vi "Main.vi"(8 "error in (no error)":errorcluster, 11 "ModuleAdmin":refnum<class "ModuleAdmin.lvclass">) -> ()   [LabVIEW 2018, in "DigitizerPlugins.lvlib"]
uses:
  DigitizerPlugins.lvlib
  <userlib>/NIST/ModuleAdminLib/ModuleAdmin/ModuleAdmin.lvclass
  C:/Program Files/National Instruments/LabVIEW 2018/user.lib/NIST/ModuleAdminLib/ModuleAdminBase/ModuleAdminBase.lvclass
  DigitizerShared/clStopArgument.ctl
  DigitizerBaseClass/DigitizerBase.lvclass
  C:/Program Files/National Instruments/LabVIEW 2018/user.lib/NIST/BaseClasses/BasePlugin_class/BasePlugin.lvclass
  <userlib>/NIST/ModuleAdminLib/ModuleAdmin/ModuleAdmin.lvclass/ModuleAdmin.ctl
  <userlib>/NIST/BaseClasses/BasePlugin_class/BasePlugin.lvclass/BasePlugin.ctl
  DigitizerBaseClass/DigitizerBase.lvclass/DigitizerBase.ctl
  DigitizerBaseClass/Typedefs/Channel.ctl
  DigitizerBaseClass/Typedefs/Acquisition.ctl
  DigitizerBaseClass/Typedefs/Trigger.ctl
  DigitizerBaseClass/Typedefs/TrigSource.ctl
  <vilib>/Utility/error.llb/DialogType.ctl
  <userlib>/NIST/ModuleAdminLib/ModuleAdmin/Accessors/Read ShowPanel_.vi
  <userlib>/NIST/ModuleAdminLib/ModuleAdmin/Accessors/Write ShowPanel_.vi
  <userlib>/NIST/BaseClasses/BasePlugin_class/Accessors/Write PluginIniFilePath.vi
  <userlib>/NIST/BaseClasses/BasePlugin_class/Accessors/Read PluginIniFilePath.vi
  DigitizerBaseClass/Accessors/Read Channels.vi
  DigitizerBaseClass/Accessors/Write Channels.vi
  DigitizerBaseClass/Accessors/Read Acquisition.vi
  DigitizerBaseClass/Accessors/Write Acquisition.vi
  DigitizerBaseClass/Accessors/Read Trigger.vi
  DigitizerBaseClass/Accessors/Write Trigger.vi
  DigitizerBaseClass/Accessors/Read Waveforms.vi
  <userlib>/NIST/ModuleAdminLib/ModuleAdmin/Accessors/Read CloneRegRef.vi
  <extravilib>/ChannelInstances/Tag-bool/Read With Abort.vi
  <extravilib>/ChannelInstances/Tag-bool/Write With Abort.vi
  <extravilib>/ChannelInstances/Tag-bool/Instantiate.vi
  <extravilib>/ChannelInstances/Tag-bool/EndpointRead.vi
  <vilib>/Utility/error.llb/Error Cluster From Error Code.vi
  <extravilib>/ChannelInstances/Tag-bool/Endpoint.vi
  <vilib>/ErrorRing/Error Ring.xnode
  <userlib>/NIST/ModuleAdminLib/CloneRegistration/CloneRegistration.lvclass
  DigitizerShared/DigitizerShared.lvlib
  <userlib>/NIST/BaseClasses/Object_class/BaseObject.lvclass
  <userlib>/NIST/ModuleAdminLib/ModuleAdmin.lvlib
  <extravilib>/ChannelInstances/Tag-bool.lvlib
panel:
  out "error out":errorcluster
  # "This is the template for your cloneable module.\nYou should modifiy this to perform the functionality\nthat you want it to perform"
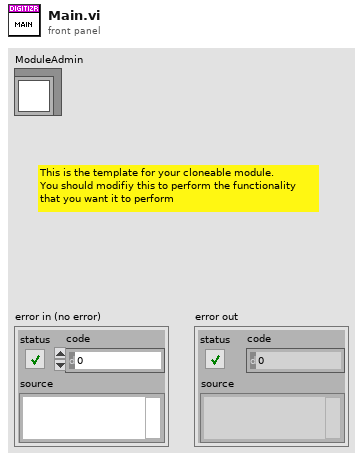
[diagram p1: front panel]
types:
  T1 = typedef "DigitizerShared.lvlib/clRequestEvents.ctl" = cluster{"StopRequest":refnum<user-event>, "PathToINI":refnum<user-event>, " LoadPlugin":refnum<user-event>, "ShowPanel":refnum<user-event>, "PrefDlg":refnum<user-event>, "ReadChannels":refnum<user-event>, "WriteChannels":refnum<user-event>, "ConfigChannels":refnum<user-event>, "ReadAcq":refnum<user-event>, "WriteAcq":refnum<user-event>, "ConfigAcq":refnum<user-event>, "ReadTriggers":refnum<user-event>, "WriteTriggers":refnum<user-event>, "ConfigTriggers":refnum<user-event>, "FetchWfrm":refnum<user-event>, "ReadWfrm":refnum<user-event>, "Initialize":refnum<user-event>, "Abort":refnum<user-event>, "ReadSyncInfo":refnum<user-event>, "WriteSyncInfo":refnum<user-event>, "Close":refnum<user-event>}
  T2 = typedef "DigitizerShared.lvlib/clBroadcastEvents.ctl" = cluster{"DidInit":refnum<user-event>, "StatusUpdate":refnum<user-event>, "ErrorReport":refnum<user-event>, "DidStop":refnum<user-event>, "PathToINI":refnum<user-event>, "Channels":refnum<user-event>, "Acq":refnum<user-event>, "Trigger":refnum<user-event>, "Waveforms":refnum<user-event>}
  T3 = typedef "DigitizerShared.lvlib/clStopArgument.ctl" = cluster{"Exit via Stop Module Req?":bool, "Wait for Module to stop?":bool, "ModuleAdmin":refnum<class "ModuleAdmin.lvclass">}
  T4 = enum32{"Invalid", "Standard", "Closed", "Hidden", "Minimized", "Maximized"}
  T5 = typedef "DigitizerPlugins.lvlib/DigitizerBase.lvclass/Channel.ctl" = cluster{"Name":string, "Enabled":bool, "InputImpedance":dbl, "Coupling":enum16{"AC", "DC", "Gnd"}, "Offset":dbl, "Range":dbl}
  T6 = typedef "DigitizerPlugins.lvlib/DigitizerBase.lvclass/Acquisition.ctl" = cluster{"SampleRate":dbl, "RecordSize":i32, "NumRecords":i32, "SampleMode":i32, "Timeout (ms)":i32}
  T7 = typedef "DigitizerPlugins.lvlib/DigitizerBase.lvclass/Trigger.ctl" = cluster{"Source":string, "Delay":dbl, "Holdoff":dbl, "PretriggerSamples":i32, "Sources":T8[]}
  T8 = typedef "DigitizerPlugins.lvlib/DigitizerBase.lvclass/TrigSource.ctl" = cluster{"Name":string, "Coupling":enum16{"AC", "DC", "HF Reject", "LF Reject", "Noise Reject"}, "Hysteresis":dbl, "Level":dbl, "Slope":enum16{"Positive", "Negative"}, "Type":enum16{"Edge", "Width", "Runt", "Glitch", "TV", "Window"}}
  T9 = typedef "Tag-bool.lvlib/))Channel.ctl" = refnum<queue>
  T10 = typedef "DialogType.ctl" = u16
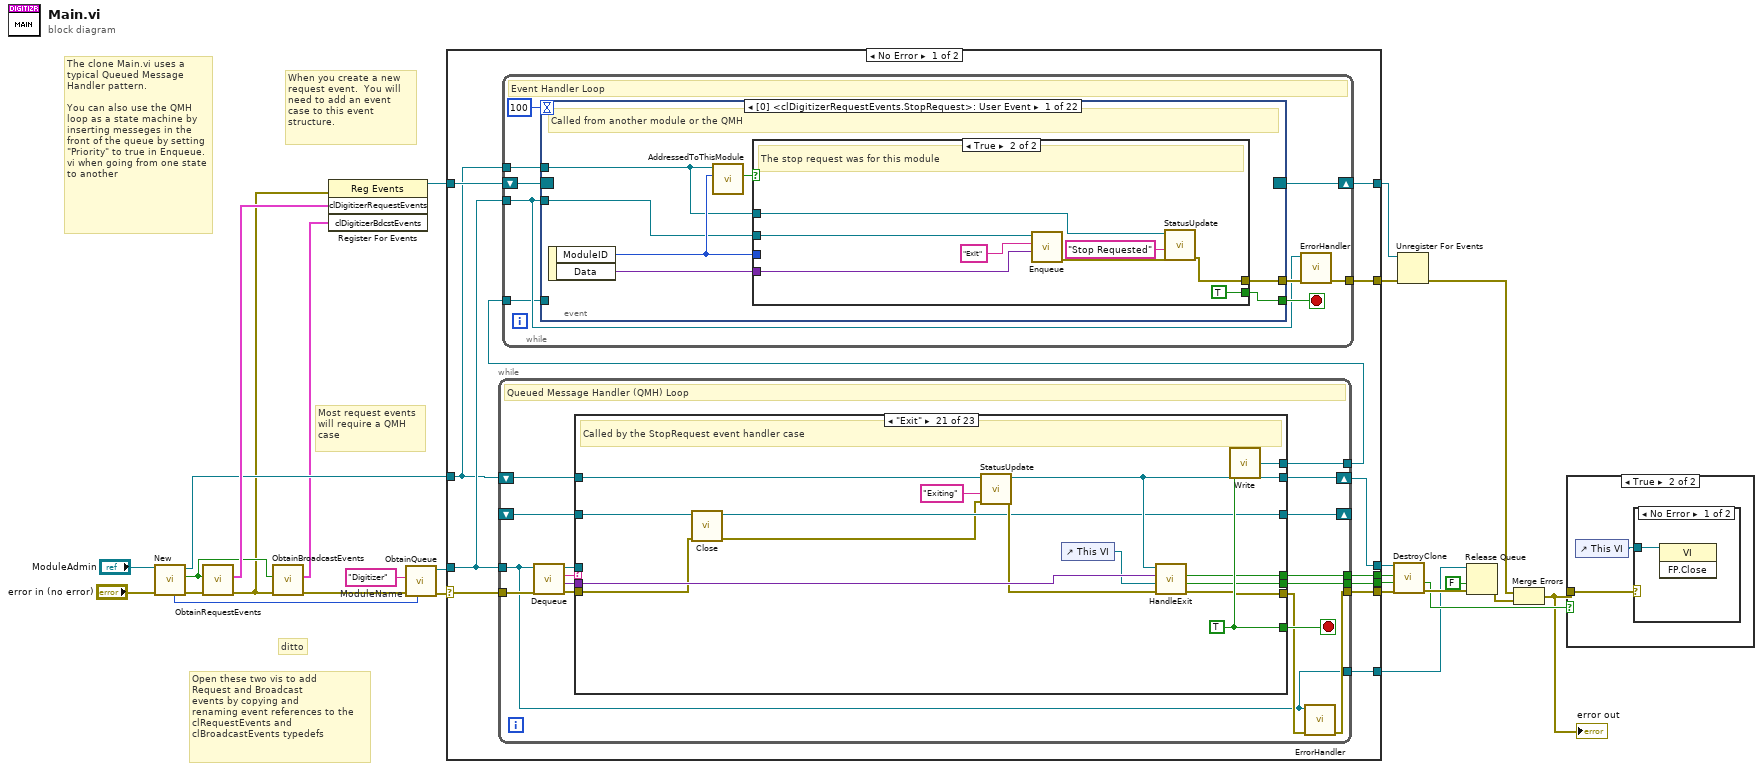
[diagram p0: block diagram]
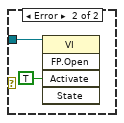
[diagram p3: hidden frame]
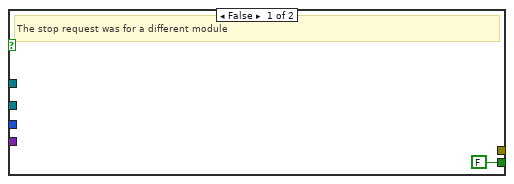
[diagram p4: hidden frame]
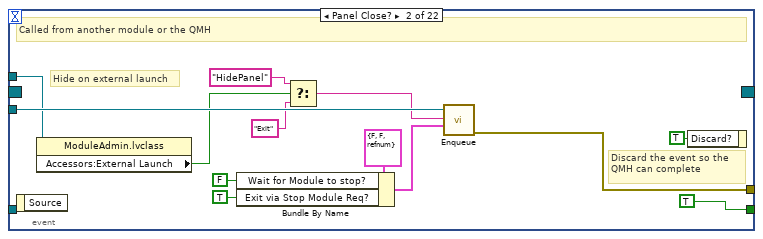
[diagram p5: hidden frame]
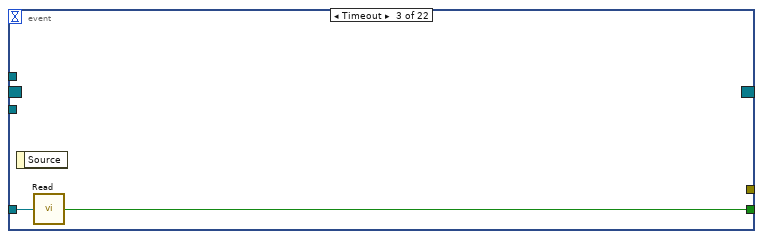
[diagram p6: hidden frame]
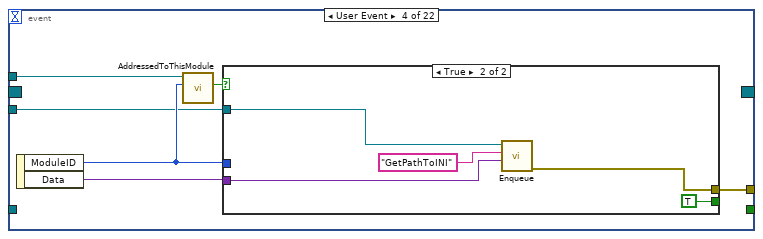
[diagram p7: hidden frame]
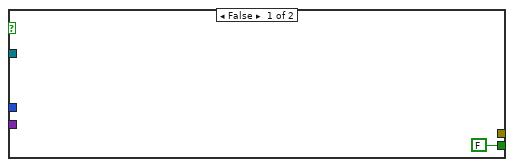
[diagram p8: hidden frame]
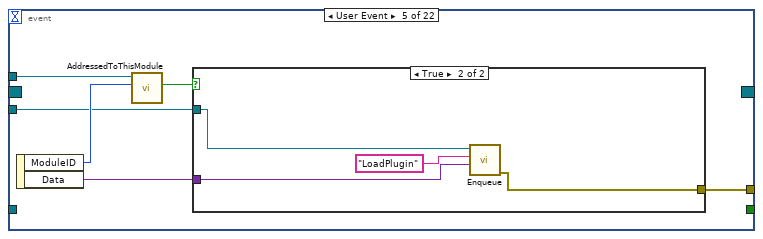
[diagram p9: hidden frame]
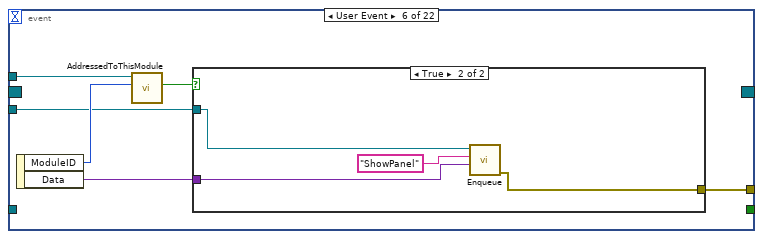
[diagram p11: hidden frame]
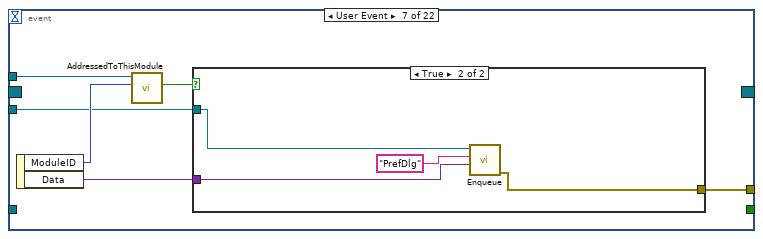
[diagram p13: hidden frame]
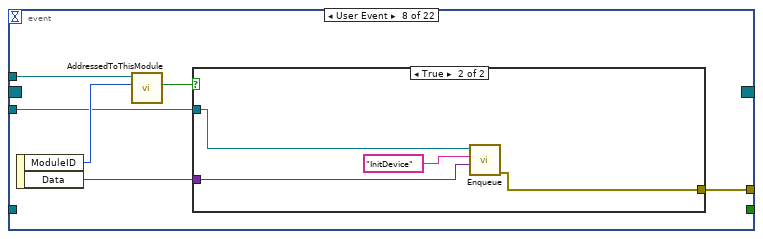
[diagram p15: hidden frame]
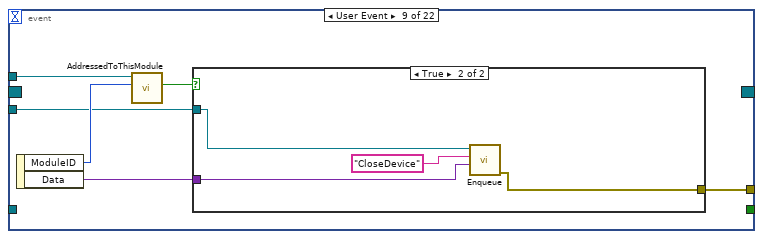
[diagram p17: hidden frame]
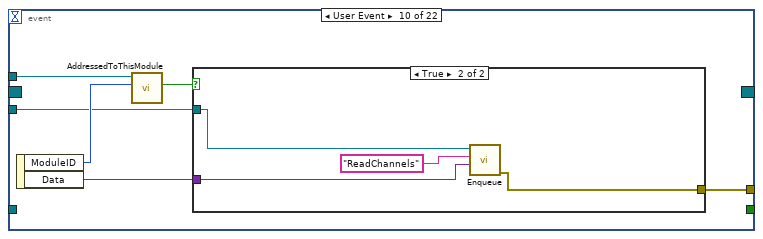
[diagram p19: hidden frame]
diagram:
  w1 = "Digitizer"  # ModuleName
  # "The clone Main.vi uses a typical Queued Message Handler pattern.  \n\nYou can also use the QMH loop as a state machine by inserting messeges in the front of the queue by setting \"Priority\" to true in Enqueue.vi when going from one state to another"
  # "Open these two vis to add\nRequest and Broadcast \nevents by copying and \nrenaming event references to the \nclRequestEvents and \nclBroadcastEvents typedefs"
  # "ditto"
  # "Most request events\nwill require a QMH\ncase"
  # "When you create a new request event.  You will need to add an event case to this event structure."
  n1 = call <userlib>:"New.vi"("error in (no error)"="error in (no error)", "ModuleAdmin"="ModuleAdmin") -> ("error out"=w25:errorcluster, "First?"=w19:bool, "ModuleAdmin"=w21:refnum<class "ModuleAdmin.lvclass">, "Module ID"=w2:i32)  [unwired: 6 in]
  n2 = call "ObtainRequestEvents.vi"("error in (no error)"=w25, "CreateNew (F)"=w19) -> ("error out"=w18:errorcluster, "clDigitizerRequestEvents"=w24:T1)  [unwired: 8 in]
  n3 = call "ObtainBroadcastEvents.vi"("error in (no error)"=w18, "CreateNew? (F)"=w19) -> ("error out"=w20:errorcluster, "clDigitizerBdcstEvents"=w17:T2)  [unwired: 8 in]
  n4 = register-events(error in=w18, w24, w17) -> (reference out=w16:refnum<event-registration>)  [unwired: 1 in, 1 out]
  n5 = call "ObtainQueue.vi"("ModuleID"=w2, "error in (no error)"=w20, "ModuleName"=w1) -> ("error out"=w23:errorcluster, "MessageQueue"=w22:refnum<queue>)  [unwired: 7 in]
  n6 = case shown="No Error" w23 {
    selector: w23 -> [w39 w631]
    tunnel: w22 -> [w37 w623]
    tunnel: w21 -> [w35 w628]
    tunnel: [w38 w629] -> w15
    tunnel: w16 -> [w36 w624]
    tunnel: [w34 w627] -> w13
    tunnel: [w33 _] -> w12
    tunnel: [w32 _] -> w11
    tunnel: [w31 _] -> w8
    tunnel: [w30 w624] -> w7
    tunnel: [w29 w623] -> w4
    frame No Error {
      n7 = while {
        tunnel: w37 -> [w274]
        tunnel: w39 -> [w286]
        tunnel: [w279] -> w38
        tunnel: [w281] -> w33
        tunnel: [w280] -> w32
        shift-right: [w277] -> _
        shift-left: _ -> [w276]
        shift-right: [w275] -> w34
        shift-left: w35 -> [w282]
        tunnel: [w274] -> w29
        tunnel: [w273] -> w28
        stop <- w287 stop-if-true
        # "Queued Message Handler (QMH) Loop"
        n8 = call "Dequeue.vi"("error in (no error)"=w286, "MessageQueue"=w274) -> ("error out"=w285:errorcluster, "Message Data"=w283:variant, "Message"=w284:string, "MessageQueue"=w272:refnum<queue>)  [unwired: 6 in]
        n9 = case shown="\"Exit\"" w284 {
          selector: w284 -> [_ _ _ _ _ _ _ _ _ _ _ _ _ _ _ _ _ _ _ _ _ _ w611]
          tunnel: [_ _ _ _ _ _ _ _ _ _ _ _ _ _ _ _ _ _ _ _ w581 _ _] -> w287
          tunnel: w282 -> [w308 w325 w333 w380 w383 w394 w399 w414 w428 w433 w448 w462 w467 w484 w491 w502 w517 w530 w546 w558 w575 w585 w614]
          tunnel: [w297 w318 w334 w381 w386 w388 w396 w408 w423 w430 w442 w457 w464 w481 w485 w500 w515 w521 w537 w553 w580 w586 w610] -> w278
          tunnel: w285 -> [_ w328 w343 w376 w387 w392 w406 w411 w427 w440 w443 w461 w474 w478 w488 w504 w519 w528 w543 w557 w569 w594 _]
          tunnel: w283 -> [_ w327 w345 _ _ _ w407 _ _ w441 _ _ w475 w479 _ _ _ _ _ _ w579 w593 _]
          tunnel: [_ _ _ _ _ _ _ _ _ _ _ _ _ _ _ _ _ _ _ _ w577 _ _] -> w281
          tunnel: [_ _ _ _ _ _ _ _ _ _ _ _ _ _ _ _ _ _ _ _ w576 _ _] -> w280
          tunnel: [refnum<class "DigitizerBase.lvclass"> refnum ("MyPlugins.lvlib:MyPluginsBase.lvclass") w317 w331 w377 w384 w390 w402 w409 w425 w436 w445 w459 w470 w477 w486 w501 w516 w523 w541 w555 w570 w584 w608] -> w277
          tunnel: w276 -> [_ w317 w332 w379 w385 w395 w404 w412 w429 w438 w446 w463 w472 w480 w489 w505 w520 w526 w545 w556 w571 w584 w608]
          tunnel: [w288 w324 w329 w374 w383 w389 w398 w413 w424 w432 w447 w458 w466 w483 w490 w499 w514 w522 w539 w559 w574 w583 w607] -> w275
          tunnel: [_ _ _ _ _ _ _ _ _ _ _ _ _ _ _ _ _ _ _ _ w567 _ _] -> w273
          tunnel: w272 -> [_ _ _ _ _ _ _ _ _ _ _ _ _ _ _ _ _ _ _ _ _ w582 _]
          frame "Initialize" {
            # "Initialize is always called after ObtainQueue.vi is run"
            n10 = property class="ModuleAdmin.lvclass"(reference=w308) -> (reference out=w294:refnum<class "ModuleAdmin.lvclass">, error out=w305:errorcluster, "Accessors:Module ID"=w296:i32, "Accessors:ShowPanel_"=w291:bool, "Accessors:External Launch"=w290:bool, "Accessors:ModuleName"=w292:string)  [unwired: 1 in]
            n11 = Compound Arithmetic op=OR(w291, invert w290) -> (w289:bool)
            n12 = Select(t=T4."Standard" ("Front Panel Window:State"), s=w289, f=T4."Hidden" ("Front Panel Window:State")) -> (s? t:f=w301:T4)
            n13 = invoke class="VI" method="FP.Open"(error in=w305, "State"=w301) -> (error out=w304:errorcluster)  [unwired: 3 in, 4 out]
            n14 = call <userlib>:"ModuleName.vi"("Name"=w292, "ModuleID"=w296) -> ("ModuleName"=w300:string)  [unwired: 9 in]
            n15 = property class="VI"(error in=w304, "Front Panel.Title"=w300) -> (reference out=w307:refnum<vi>, error out=w306:errorcluster)  [unwired: 1 in]
            n16 = invoke class="VI" method="FP.Center"(reference=w307, error in=w306) -> (error out=w295:errorcluster)  [unwired: 1 in, 2 out]
            n17 = case shown="True" w290 {
              tunnel: [w309 w315] -> w298
              tunnel: [w310 w312] -> w288
              tunnel: w295 -> [w309 w314]
              tunnel: w294 -> [w310 w311]
              frame False {
              }
              frame True {
                n18 = call <userlib>:"WaitOnModuleSync.vi"("error in (no error)"=w314, "ModuleAdmin"=w311) -> ("error out"=w316:errorcluster, "ModuleAdmin"=w313:refnum<class "ModuleAdmin.lvclass">)  [unwired: 8 in]
                n19 = call <userlib>:"WaitOnEventSync.vi"("error in (no error)"=w316, "ModuleAdmin"=w313) -> ("error out"=w315:errorcluster, "ModuleAdmin"=w312:refnum<class "ModuleAdmin.lvclass">)  [unwired: 8 in]
              }
            }
            n20 = call "DidInit.vi"("Init?"=TRUE, "error in (no error)"=w298, "ModuleAdmin"=w288) -> ("error out"=w297:errorcluster)  [unwired: 8 in]
          }
          frame "ShowPanel" {
            # "The frontpanel can be shown or hidden"
            n21 = Variant To Data(error in=w328, type=TRUE, Variant=w327) -> (data=w320:bool, error out=w323:errorcluster)
            n22 = Select(t=T4."Standard" ("Front Panel Window:State"), s=w320, f=T4."Hidden" ("Front Panel Window:State")) -> (s? t:f=w319:T4)
            n23 = property class="VI"(error in=w323, "FP.State"=w319) -> (error out=w318:errorcluster)  [unwired: 1 in, 1 out]
            n24 = property class="ModuleAdmin.lvclass"(reference=w325, "Accessors:ShowPanel_"=w320) -> (reference out=w324:refnum<class "ModuleAdmin.lvclass">)  [unwired: 1 in, 1 out]
          }
          frame "LoadPlugin" {
            # "Dynamically oads and initializes a plugin from the .ini file"
            n25 = Variant To Data(error in=w343, type=path "", Variant=w345) -> (data=w330:path, error out=w342:errorcluster)
            n26 = call <userlib>:"GetPathToClass.vi"("error in (no error)"=w342, "configuration file path"=w330) -> ("error IO"=w338:errorcluster, "PathToClass"=w341:path)  [unwired: 8 in]
            n27 = Current VI's Path() -> (path=w340:path)
            n28 = Build Path(base path=w340, name or relative path=w341) -> (appended path=w339:path)
            n29 = call <vilib>:"Check if File or Folder Exists.vi"("error in (no error)"=w338, "path"=w339) -> ("error out"=w335:errorcluster, "file or folder exists?"=w337:bool, "dup path"=w336:path)  [unwired: 7 in]
            n30 = case shown="True" w337 {
              tunnel: w336 -> [w349 w366]
              tunnel: w335 -> [_ w373]
              tunnel: [w348 w368] -> w334
              tunnel: w333 -> [w346 w363]
              tunnel: w332 -> [w347 _]
              tunnel: [w347 w359] -> w331
              tunnel: w330 -> [_ w364]
              tunnel: [w346 w362] -> w329
              frame False {
                n31 = Path To String(path=w349) -> (string=w350:string)
                n32 = xnode "Error Ring"("parameter 0"=w350) -> ("error out"=w348:errorcluster)
              }
              frame True {
                n33 = call-dynamic "LoadClassFromFile.vi"("error in (no error)"=w373, "class path"=w366, "reference in"=refnum<class "DigitizerBase.lvclass"> refnum ("MyPlugins.lvlib:MyPluginsBase.lvclass")) -> ("error out"=w365:errorcluster, "reference out"=w367:refnum<class "DigitizerBase.lvclass">)  [unwired: 7 in]
                n34 = property class="DigitizerBase.lvclass"(reference=w367, error in=w365, "Accessors:PluginIniFilePath"=w364) -> (reference out=w361:refnum<class "DigitizerBase.lvclass">, error out=w360:errorcluster)
                n35 = Path To String(path=w366) -> (string=w370:string)
                n36 = Format Into String(format string="Plugin %s loaded ", w370) -> (resulting string=w369:string)  [unwired: 2 in, 1 out]
                n37 = call-dynamic "DefaultFromIni.vi"("error in (no error)"=w360, "MyPluginsBase in"=w361) -> ("error out"=w358:errorcluster, "MyPluginsBase out"=w359:refnum<class "DigitizerBase.lvclass">)  [unwired: 8 in]
                n38 = call "StatusUpdate.vi"("error in (no error)"=w358, "Status"=w369, "Module"=w363) -> ("error out"=w368:errorcluster, "Module"=w362:refnum<class "ModuleAdmin.lvclass">)  [unwired: 7 in]
              }
            }
          }
          frame "GetPathToINI" {
            # "Broadcast the path to the .ini file"
            n39 = property class="DigitizerBase.lvclass"(reference=w379, error in=w376) -> (reference out=w377:refnum<class "DigitizerBase.lvclass">, error out=w375:errorcluster, "Accessors:PluginIniFilePath"=w378:path)
            n40 = property class="ModuleAdmin.lvclass"(reference=w380) -> (reference out=w374:refnum<class "ModuleAdmin.lvclass">, "Accessors:Module ID"=w382:i32)  [unwired: 1 in, 1 out]
            n41 = call "PathToINIBroadcast.vi"("error in (no error)"=w375, "PathToINI"=w378, "ModuleID"=w382) -> ("error out"=w381:errorcluster)  [unwired: 8 in]
          }
          frame "PrefDlg" {
            # "Override Base Class\\PublicMethods\\PrefDialog.vi for user editable preference dialog"
            # "Launch the modal Preferences dialog"
            n42 = call-dynamic "PrefDialog.vi"("error in (no error)"=w387, "DigitizerBase"=w385) -> ("error out"=w386:errorcluster, "DigitizerBase"=w384:refnum<class "DigitizerBase.lvclass">)  [unwired: 8 in]
          }
          frame "ReadChannels" {
            n43 = property class="DigitizerBase.lvclass"(reference=w395, error in=w392) -> (reference out=w390:refnum<class "DigitizerBase.lvclass">, error out=w391:errorcluster, "Accessors:Channels"=w393:T5[])
            n44 = call "ChannelBdcst.vi"("error in (no error)"=w391, "Channels"=w393, "Module"=w394) -> ("error out"=w388:errorcluster, "Module"=w389:refnum<class "ModuleAdmin.lvclass">)  [unwired: 7 in]
          }
          frame "WriteChannels" {
            n45 = Variant To Data(error in=w406, type=T5[] [], Variant=w407) -> (data=w403:T5[], error out=w401:errorcluster)
            n46 = property class="DigitizerBase.lvclass"(reference=w404, error in=w401, "Accessors:Channels"=w403) -> (reference out=w402:refnum<class "DigitizerBase.lvclass">, error out=w400:errorcluster)
            n47 = call "StatusUpdate.vi"("error in (no error)"=w400, "Status"="Received Channels", "Module"=w399) -> ("error out"=w396:errorcluster, "Module"=w398:refnum<class "ModuleAdmin.lvclass">)  [unwired: 7 in]
          }
          frame "ConfigChannels" {
            n48 = call-dynamic "ConfigChannels.vi"("error in (no error)"=w411, "DigitizerBase in"=w412) -> ("error out"=w410:errorcluster, "DigitizerBase out"=w409:refnum<class "DigitizerBase.lvclass">)  [unwired: 8 in]
            n49 = case shown="No Error" w410 {
              selector: w410 -> [w419 w420]
              tunnel: w414 -> [w418 w421]
              tunnel: [w416 w420] -> w408
              tunnel: [w415 w421] -> w413
              frame No Error {
                n50 = call "StatusUpdate.vi"("error in (no error)"=w419, "Status"="Channels Configured", "Module"=w418) -> ("error out"=w416:errorcluster, "Module"=w415:refnum<class "ModuleAdmin.lvclass">)  [unwired: 7 in]
              }
              frame Error {
              }
            }
          }
          frame "ReadAcq" {
            n51 = property class="DigitizerBase.lvclass"(reference=w429, error in=w427) -> (reference out=w425:refnum<class "DigitizerBase.lvclass">, error out=w426:errorcluster, "Accessors:Acquisition"=w422:T6)
            n52 = call "AcqBdcst.vi"("error in (no error)"=w426, "Acquisition"=w422, "Module"=w428) -> ("error out"=w423:errorcluster, "Module"=w424:refnum<class "ModuleAdmin.lvclass">)  [unwired: 7 in]
          }
          frame "WriteAcq" {
            n53 = Variant To Data(error in=w440, type=T6 {"SampleRate"=0.0, "RecordSize"=0, "NumRecords"=0, "SampleMode"=0, "Timeout (ms)"=0}, Variant=w441) -> (data=w437:T6, error out=w435:errorcluster)
            n54 = property class="DigitizerBase.lvclass"(reference=w438, error in=w435, "Accessors:Acquisition"=w437) -> (reference out=w436:refnum<class "DigitizerBase.lvclass">, error out=w434:errorcluster)
            n55 = call "StatusUpdate.vi"("error in (no error)"=w434, "Status"="Received Acquisition", "Module"=w433) -> ("error out"=w430:errorcluster, "Module"=w432:refnum<class "ModuleAdmin.lvclass">)  [unwired: 7 in]
          }
          frame "ConfigAcq" {
            n56 = call-dynamic "ConfigAcq.vi"("error in (no error)"=w443, "DigitizerBase in"=w446) -> ("error out"=w444:errorcluster, "DigitizerBase out"=w445:refnum<class "DigitizerBase.lvclass">)  [unwired: 8 in]
            n57 = case shown="No Error" w444 {
              selector: w444 -> [w453 w454]
              tunnel: w448 -> [w452 w455]
              tunnel: [w450 w454] -> w442
              tunnel: [w449 w455] -> w447
              frame No Error {
                n58 = call "StatusUpdate.vi"("error in (no error)"=w453, "Status"="Acquisition Configured", "Module"=w452) -> ("error out"=w450:errorcluster, "Module"=w449:refnum<class "ModuleAdmin.lvclass">)  [unwired: 7 in]
              }
              frame Error {
              }
            }
          }
          frame "ReadTriggers" {
            n59 = property class="DigitizerBase.lvclass"(reference=w463, error in=w461) -> (reference out=w459:refnum<class "DigitizerBase.lvclass">, error out=w460:errorcluster, "Accessors:Trigger"=w456:T7)
            n60 = call "TriggerBdcst.vi"("error in (no error)"=w460, "Trigger"=w456, "Module"=w462) -> ("error out"=w457:errorcluster, "Module"=w458:refnum<class "ModuleAdmin.lvclass">)  [unwired: 7 in]
          }
          frame "WriteTrigger" {
            n61 = Variant To Data(error in=w474, type=T7 {"Source"="", "Delay"=0.0, "Holdoff"=0.0, "PretriggerSamples"=0, "Sources"=[]}, Variant=w475) -> (data=w471:T7, error out=w469:errorcluster)
            n62 = property class="DigitizerBase.lvclass"(reference=w472, error in=w469, "Accessors:Trigger"=w471) -> (reference out=w470:refnum<class "DigitizerBase.lvclass">, error out=w468:errorcluster)
            n63 = call "StatusUpdate.vi"("error in (no error)"=w468, "Status"="Received Trigger", "Module"=w467) -> ("error out"=w464:errorcluster, "Module"=w466:refnum<class "ModuleAdmin.lvclass">)  [unwired: 7 in]
          }
          frame "SyncInfo" {
            n64 = call-dynamic "ConfigSyncInfo.vi"("error in (no error)"=w478, "SyncInfo"=w479, "DigitizerBase in"=w480) -> ("error out"=w476:errorcluster, "DigitizerBase out"=w477:refnum<class "DigitizerBase.lvclass">)  [unwired: 7 in]
            n65 = call "StatusUpdate.vi"("error in (no error)"=w476, "Status"="SyncInfo Configured", "Module"=w484) -> ("error out"=w481:errorcluster, "Module"=w483:refnum<class "ModuleAdmin.lvclass">)  [unwired: 7 in]
          }
          frame "ConfigTrigger" {
            n66 = call-dynamic "ConfigTrigger.vi"("error in (no error)"=w488, "DigitizerBase in"=w489) -> ("error out"=w487:errorcluster, "DigitizerBase out"=w486:refnum<class "DigitizerBase.lvclass">)  [unwired: 8 in]
            n67 = case shown="No Error" w487 {
              selector: w487 -> [w496 w497]
              tunnel: w491 -> [w495 w498]
              tunnel: [w493 w497] -> w485
              tunnel: [w492 w498] -> w490
              frame No Error {
                n68 = call "StatusUpdate.vi"("error in (no error)"=w496, "Status"="Trigger Configured", "Module"=w495) -> ("error out"=w493:errorcluster, "Module"=w492:refnum<class "ModuleAdmin.lvclass">)  [unwired: 7 in]
              }
              frame Error {
              }
            }
          }
          frame "InitDevice" {
            n69 = call-dynamic "Initialize.vi"("error in (no error)"=w504, "DigitizerBase in"=w505) -> ("error out"=w503:errorcluster, "DigitizerBase out"=w501:refnum<class "DigitizerBase.lvclass">)  [unwired: 8 in]
            n70 = case shown="No Error" w503 {
              selector: w503 -> [w510 w511]
              tunnel: w502 -> [w509 w512]
              tunnel: [w507 w511] -> w500
              tunnel: [w506 w512] -> w499
              frame No Error {
                n71 = call "StatusUpdate.vi"("error in (no error)"=w510, "Status"="Digitizer Initialized", "Module"=w509) -> ("error out"=w507:errorcluster, "Module"=w506:refnum<class "ModuleAdmin.lvclass">)  [unwired: 7 in]
              }
              frame Error {
              }
            }
          }
          frame "CloseDevice" {
            n72 = call-dynamic "Close.vi"("error in (no error)"=w519, "DigitizerBase in"=w520) -> ("error out"=w518:errorcluster, "DigitizerBase out"=w516:refnum<class "DigitizerBase.lvclass">)  [unwired: 8 in]
            n73 = call "StatusUpdate.vi"("error in (no error)"=w518, "Status"="Digitizer Closed", "Module"=w517) -> ("error out"=w515:errorcluster, "Module"=w514:refnum<class "ModuleAdmin.lvclass">)  [unwired: 7 in]
          }
          frame "FetchWfrms" {
            n74 = call "StatusUpdate.vi"("error in (no error)"=w528, "Status"="Beginning Fetch", "Module"=w530) -> ("error out"=w527:errorcluster, "Module"=w524:refnum<class "ModuleAdmin.lvclass">)  [unwired: 7 in]
            n75 = call-dynamic "FetchAllDbl.vi"("error in (no error)"=w527, "DigitizerBase in"=w526) -> ("error out"=w525:errorcluster, "DigitizerBase out"=w523:refnum<class "DigitizerBase.lvclass">)  [unwired: 8 in]
            n76 = case shown="No Error" w525 {
              selector: w525 -> [_ w535]
              tunnel: w524 -> [w534 w536]
              tunnel: [w532 w536] -> w522
              tunnel: [w531 w535] -> w521
              frame No Error {
                n77 = call "StatusUpdate.vi"("Status"="Fetch Complete", "Module"=w534) -> ("error out"=w531:errorcluster, "Module"=w532:refnum<class "ModuleAdmin.lvclass">)  [unwired: 8 in]
              }
              frame Error {
              }
            }
          }
          frame "ReadWfrms" {
            n78 = property class="DigitizerBase.lvclass"(reference=w545, error in=w543) -> (reference out=w541:refnum<class "DigitizerBase.lvclass">, error out=w542:errorcluster, "Accessors:Waveforms"=w544:variant)
            n79 = call "WfrmBdcst.vi"("error in (no error)"=w542, "Waveforms"=w544, "Module"=w546) -> ("error out"=w538:errorcluster, "Module"=w540:refnum<class "ModuleAdmin.lvclass">)  [unwired: 7 in]
            n80 = case shown="No Error" w538 {
              selector: w538 -> [_ w551]
              tunnel: w540 -> [w550 w552]
              tunnel: [w548 w552] -> w539
              tunnel: [w547 w551] -> w537
              frame No Error {
                n81 = call "StatusUpdate.vi"("Status"="Read Complete", "Module"=w550) -> ("error out"=w547:errorcluster, "Module"=w548:refnum<class "ModuleAdmin.lvclass">)  [unwired: 8 in]
              }
              frame Error {
              }
            }
          }
          frame "Abort" {
            n82 = call-dynamic "Abort.vi"("error in (no error)"=w557, "DigitizerBase in"=w556) -> ("error out"=w554:errorcluster, "DigitizerBase out"=w555:refnum<class "DigitizerBase.lvclass">)  [unwired: 8 in]
            n83 = case shown="Error" w554 {
              selector: w554 -> [w560 w565]
              tunnel: w558 -> [w564 w566]
              tunnel: [w562 w566] -> w559
              tunnel: [w561 w565] -> w553
              frame No Error {
                n84 = call "StatusUpdate.vi"("error in (no error)"=w560, "Status"="Abort Complete", "Module"=w564) -> ("error out"=w561:errorcluster, "Module"=w562:refnum<class "ModuleAdmin.lvclass">)  [unwired: 7 in]
              }
              frame Error {
              }
            }
          }
          frame "Exit" {
            w581 = TRUE
            # "Called by the StopRequest event handler case"
            n85 = call-dynamic "Close.vi"("error in (no error)"=w569, "DigitizerBase in"=w571) -> ("error out"=w568:errorcluster, "DigitizerBase out"=w570:refnum<class "DigitizerBase.lvclass">)  [unwired: 8 in]
            n86 = call "StatusUpdate.vi"("error in (no error)"=w568, "Status"="Exiting", "Module"=w575) -> ("error out"=w572:errorcluster, "Module"=w574:refnum<class "ModuleAdmin.lvclass">)  [unwired: 7 in]
            n87 = control-ref of="This VI"() -> (w578:refnum<vi>)
            n88 = call "HandleExit.vi"("error in (no error)"=w572, "VI Refnum"=w578, "StopArgument"=w579, "ModuleAdmin"=w574) -> ("error out"=w580:errorcluster, "Exit via Stop Module Req?"=w576:bool, "WaitForStop?"=w577:bool)  [unwired: 5 in]
            n89 = call <extravilib>:"Write.vi"("element"=w581) -> ("channel"=w567:T9)  [unwired: 1 out]
          }
          frame "Error" {
            # "Handle any errors"
            n90 = property class="ModuleAdmin.lvclass"(reference=w585) -> (reference out=w583:refnum<class "ModuleAdmin.lvclass">, "Accessors:External Launch"=w589:bool, "Accessors:Module ID"=w587:i32)  [unwired: 1 in, 1 out]
            n91 = Variant To Data(error in=w594, type=errorcluster {"status"=FALSE, "code"=0, "source"=""} ("error constant"), Variant=w593) -> (data=w588:errorcluster, error out=w591:errorcluster)
            n92 = call "ReportError.vi"("error in (no error)"=w591, "ErrorReported"=w588, "ModuleID"=w587) -> ("error out"=w590:errorcluster)  [unwired: 8 in]
            n93 = case shown="True" w589 {
              tunnel: w590 -> [w598 w601]
              tunnel: w588 -> [w597 _]
              tunnel: [w596 w600] -> w586
              tunnel: w585 -> [w595 _]
              tunnel: w582 -> [_ w599]
              frame False {
                # "Todo:  Add an event to ask the user\nIf the module should stop or continue"
                # "Stand alone: now, force an exit"
                n94 = call <vilib>:"Simple Error Handler.vi"("error in (no error)"=w597) -> ()  [unwired: 4 in, 5 out]
                n95 = call "StopRequest.vi"("error in (no error)"=w598, "ModuleAdmin"=w595) -> ("error out"=w596:errorcluster)  [unwired: 8 in, 1 out]
              }
              frame True {
                # "Externally launched modules only broadcast the error msg"
                n96 = case shown="No Error" w601 {
                  selector: w601 -> [w602 w606]
                  tunnel: [w602 _] -> w600
                  tunnel: w599 -> [_ w605]
                  frame No Error {
                  }
                  frame Error {
                    n97 = call "Enqueue.vi"("Priority (F)"=TRUE, "error in (no error)"=w606, "Message"="Exit", "MessageQueue"=w605) -> ()  [unwired: 6 in, 2 out]
                  }
                }
              }
            }
          }
          frame Default {
            # "Called only if a message was queued and no QMH case was created"
            n98 = property class="ModuleAdmin.lvclass"(reference=w614) -> (reference out=w607:refnum<class "ModuleAdmin.lvclass">, "Accessors:Module ID"=w613:i32, "Accessors:ModuleName"=w609:string)  [unwired: 1 in, 1 out]
            n99 = call <userlib>:"ModuleName.vi"("Name"=w609, "ModuleID"=w613) -> ("ModuleName"=w612:string)  [unwired: 9 in]
            n100 = xnode "Error Ring"("parameter 0"=w611, "parameter 1"=w612) -> ("error out"=w610:errorcluster)
          }
        }
        n101 = call "ErrorHandler.vi"("error in (no error)"=w278, "MessageQueue"=w274) -> ("error out"=w279:errorcluster)  [unwired: 8 in, 1 out]
      }
      n102 = while {
        tunnel: w37 -> [w42]
        shift-right: [w46] -> w30
        shift-left: w36 -> [w47]
        tunnel: w35 -> [w45]
        tunnel: [w43] -> w31
        tunnel: w28 -> [w40]
        stop <- w48 stop-if-true
        # "Event Handler Loop"
        n103 = event shown="[0] <clDigitizerRequestEvents.StopRequest>: User Event" {
          selector: w47 -> [_ _ _ _ _ _ _ _ _ _ _ _ _ _ _ _ _ _ _ _ _ _]
          dyn-events: [_ _ _ _ _ _ _ _ _ _ _ _ _ _ _ _ _ _ _ _ _ _] -> w46
          timeout: 100 -> [_ _ _ _ _ _ _ _ _ _ _ _ _ _ _ _ _ _ _ _ _ _]
          tunnel: w42 -> [w53 w77 _ w82 w93 w103 w113 w123 w133 w143 w153 w163 w173 w183 w193 w203 w213 w223 w233 w243 w253 w263]
          tunnel: [w52 TRUE w78 _ _ _ _ _ _ _ _ _ _ _ _ _ _ _ _ _ _ _] -> w48
          tunnel: w45 -> [w49 w71 _ w81 w97 w107 w117 w127 w137 w147 w157 w167 w177 w187 w197 w207 w217 w227 w237 w247 w257 w267]
          tunnel: [w51 w75 _ w80 w94 w104 w114 w124 w134 w144 w154 w164 w174 w184 w194 w204 w214 w224 w234 w244 w254 w264] -> w44
          tunnel: w40 -> [_ _ w79 _ _ _ _ _ _ _ _ _ _ _ _ _ _ _ _ _ _ _]
          event User Event {
            # "Called from another module or the QMH"
            n104 = event-data() -> ("ModuleID"=w54:i32, "Data"=w50:variant)  [unwired: 1 in]
            n105 = call <userlib>:"AddressedToThisModule.vi"("ModuleID"=w54, "ModuleAdmin"=w49) -> ("AddressedToThisInstance?"=w55:bool)  [unwired: 8 in, 1 out]
            n106 = case shown="True" w55 {
              tunnel: w54 -> [_ _]
              tunnel: w53 -> [_ w64]
              tunnel: [FALSE TRUE] -> w52
              tunnel: [_ w59] -> w51
              tunnel: w50 -> [_ w61]
              tunnel: w49 -> [_ w57]
              frame False {
                # "The stop request was for a different module"
              }
              frame True {
                # "The stop request was for this module"
                n107 = call "Enqueue.vi"("Message Data"=w61, "Message"="Exit", "MessageQueue"=w64) -> ("error out"=w60:errorcluster)  [unwired: 7 in, 1 out]
                n108 = call "StatusUpdate.vi"("error in (no error)"=w60, "Status"="Stop Requested", "Module"=w57) -> ("error out"=w59:errorcluster)  [unwired: 7 in, 1 out]
              }
            }
          }
          event Panel Close? {
            # "Hide on external launch"
            # "Discard the event so the QMH can complete"
            # "Called from another module or the QMH"
            n109 = event-data() -> ()  [unwired: 1 in, 1 out]
            n110 = property class="ModuleAdmin.lvclass"(reference=w71) -> ("Accessors:External Launch"=w66:bool)  [unwired: 1 in, 2 out]
            n111 = Bundle By Name(cluster=T3 {"Exit via Stop Module Req?"=FALSE, "Wait for Module to stop?"=FALSE, "ModuleAdmin"=refnum} ("Stop Argument"), "Wait for Module to stop?"=FALSE, "Exit via Stop Module Req?"=TRUE) -> (w72:T3)
            n112 = Select(t="HidePanel", s=w66, f="Exit" ("Message")) -> (s? t:f=w68:string)
            n113 = call "Enqueue.vi"("Message Data"=w72, "Message"=w68, "MessageQueue"=w77) -> ("error out"=w75:errorcluster)  [unwired: 7 in, 1 out]
            n114 = event-data("Discard?"=TRUE) -> ()  [unwired: 1 in, 1 out]
          }
          event Timeout {
            n115 = event-data() -> ()  [unwired: 1 in, 1 out]
            n116 = call <extravilib>:"Read.vi"("channel"=w79) -> ("element"=w78:bool)  [unwired: 1 in, 1 out]
          }
          event User Event {
            n117 = event-data() -> ("ModuleID"=w83:i32, "Data"=w84:variant)  [unwired: 1 in]
            n118 = call <userlib>:"AddressedToThisModule.vi"("ModuleID"=w83, "ModuleAdmin"=w81) -> ("AddressedToThisInstance?"=w85:bool)  [unwired: 8 in, 1 out]
            n119 = case shown="True" w85 {
              tunnel: w83 -> [_ _]
              tunnel: w82 -> [_ w91]
              tunnel: [FALSE TRUE] -> _
              tunnel: [_ w89] -> w80
              tunnel: w84 -> [_ w87]
              frame False {
                # "The stop request was for a different module"
              }
              frame True {
                # "The stop request was for this module"
                n120 = call "Enqueue.vi"("Message Data"=w87, "Message"="GetPathToINI", "MessageQueue"=w91) -> ("error out"=w89:errorcluster)  [unwired: 7 in, 1 out]
              }
            }
          }
          event User Event {
            n121 = event-data() -> ("ModuleID"=w96:i32, "Data"=w92:variant)  [unwired: 1 in]
            n122 = call <userlib>:"AddressedToThisModule.vi"("ModuleID"=w96, "ModuleAdmin"=w97) -> ("AddressedToThisInstance?"=w95:bool)  [unwired: 8 in, 1 out]
            n123 = case shown="True" w95 {
              tunnel: [_ w98] -> w94
              tunnel: w93 -> [_ w101]
              tunnel: w92 -> [_ w99]
              frame False {
              }
              frame True {
                n124 = call "Enqueue.vi"("Message Data"=w99, "Message"="LoadPlugin", "MessageQueue"=w101) -> ("error out"=w98:errorcluster)  [unwired: 7 in, 1 out]
              }
            }
          }
          event User Event {
            n125 = event-data() -> ("ModuleID"=w106:i32, "Data"=w102:variant)  [unwired: 1 in]
            n126 = call <userlib>:"AddressedToThisModule.vi"("ModuleID"=w106, "ModuleAdmin"=w107) -> ("AddressedToThisInstance?"=w105:bool)  [unwired: 8 in, 1 out]
            n127 = case shown="True" w105 {
              tunnel: [_ w108] -> w104
              tunnel: w103 -> [_ w111]
              tunnel: w102 -> [_ w109]
              frame False {
              }
              frame True {
                n128 = call "Enqueue.vi"("Message Data"=w109, "Message"="ShowPanel", "MessageQueue"=w111) -> ("error out"=w108:errorcluster)  [unwired: 7 in, 1 out]
              }
            }
          }
          event User Event {
            n129 = event-data() -> ("ModuleID"=w116:i32, "Data"=w112:variant)  [unwired: 1 in]
            n130 = call <userlib>:"AddressedToThisModule.vi"("ModuleID"=w116, "ModuleAdmin"=w117) -> ("AddressedToThisInstance?"=w115:bool)  [unwired: 8 in, 1 out]
            n131 = case shown="True" w115 {
              tunnel: [_ w118] -> w114
              tunnel: w113 -> [_ w121]
              tunnel: w112 -> [_ w119]
              frame False {
              }
              frame True {
                n132 = call "Enqueue.vi"("Message Data"=w119, "Message"="PrefDlg", "MessageQueue"=w121) -> ("error out"=w118:errorcluster)  [unwired: 7 in, 1 out]
              }
            }
          }
          event User Event {
            n133 = event-data() -> ("ModuleID"=w126:i32, "Data"=w122:variant)  [unwired: 1 in]
            n134 = call <userlib>:"AddressedToThisModule.vi"("ModuleID"=w126, "ModuleAdmin"=w127) -> ("AddressedToThisInstance?"=w125:bool)  [unwired: 8 in, 1 out]
            n135 = case shown="True" w125 {
              tunnel: [_ w128] -> w124
              tunnel: w123 -> [_ w131]
              tunnel: w122 -> [_ w129]
              frame False {
              }
              frame True {
                n136 = call "Enqueue.vi"("Message Data"=w129, "Message"="InitDevice", "MessageQueue"=w131) -> ("error out"=w128:errorcluster)  [unwired: 7 in, 1 out]
              }
            }
          }
          event User Event {
            n137 = event-data() -> ("ModuleID"=w136:i32, "Data"=w132:variant)  [unwired: 1 in]
            n138 = call <userlib>:"AddressedToThisModule.vi"("ModuleID"=w136, "ModuleAdmin"=w137) -> ("AddressedToThisInstance?"=w135:bool)  [unwired: 8 in, 1 out]
            n139 = case shown="True" w135 {
              tunnel: [_ w138] -> w134
              tunnel: w133 -> [_ w141]
              tunnel: w132 -> [_ w139]
              frame False {
              }
              frame True {
                n140 = call "Enqueue.vi"("Message Data"=w139, "Message"="CloseDevice", "MessageQueue"=w141) -> ("error out"=w138:errorcluster)  [unwired: 7 in, 1 out]
              }
            }
          }
          event User Event {
            n141 = event-data() -> ("ModuleID"=w146:i32, "Data"=w142:variant)  [unwired: 1 in]
            n142 = call <userlib>:"AddressedToThisModule.vi"("ModuleID"=w146, "ModuleAdmin"=w147) -> ("AddressedToThisInstance?"=w145:bool)  [unwired: 8 in, 1 out]
            n143 = case shown="True" w145 {
              tunnel: [_ w148] -> w144
              tunnel: w143 -> [_ w151]
              tunnel: w142 -> [_ w149]
              frame False {
              }
              frame True {
                n144 = call "Enqueue.vi"("Message Data"=w149, "Message"="ReadChannels", "MessageQueue"=w151) -> ("error out"=w148:errorcluster)  [unwired: 7 in, 1 out]
              }
            }
          }
          event User Event {
            n145 = event-data() -> ("ModuleID"=w156:i32, "Data"=w152:variant)  [unwired: 1 in]
            n146 = call <userlib>:"AddressedToThisModule.vi"("ModuleID"=w156, "ModuleAdmin"=w157) -> ("AddressedToThisInstance?"=w155:bool)  [unwired: 8 in, 1 out]
            n147 = case shown="True" w155 {
              tunnel: [_ w158] -> w154
              tunnel: w153 -> [_ w161]
              tunnel: w152 -> [_ w159]
              frame False {
              }
              frame True {
                n148 = call "Enqueue.vi"("Message Data"=w159, "Message"="WriteChannels", "MessageQueue"=w161) -> ("error out"=w158:errorcluster)  [unwired: 7 in, 1 out]
              }
            }
          }
          event User Event {
            n149 = event-data() -> ("ModuleID"=w166:i32, "Data"=w162:variant)  [unwired: 1 in]
            n150 = call <userlib>:"AddressedToThisModule.vi"("ModuleID"=w166, "ModuleAdmin"=w167) -> ("AddressedToThisInstance?"=w165:bool)  [unwired: 8 in, 1 out]
            n151 = case shown="True" w165 {
              tunnel: [_ w168] -> w164
              tunnel: w163 -> [_ w171]
              tunnel: w162 -> [_ w169]
              frame False {
              }
              frame True {
                n152 = call "Enqueue.vi"("Message Data"=w169, "Message"="ConfigChannels", "MessageQueue"=w171) -> ("error out"=w168:errorcluster)  [unwired: 7 in, 1 out]
              }
            }
          }
          event User Event {
            n153 = event-data() -> ("ModuleID"=w176:i32, "Data"=w172:variant)  [unwired: 1 in]
            n154 = call <userlib>:"AddressedToThisModule.vi"("ModuleID"=w176, "ModuleAdmin"=w177) -> ("AddressedToThisInstance?"=w175:bool)  [unwired: 8 in, 1 out]
            n155 = case shown="True" w175 {
              tunnel: [_ w178] -> w174
              tunnel: w173 -> [_ w181]
              tunnel: w172 -> [_ w179]
              frame False {
              }
              frame True {
                n156 = call "Enqueue.vi"("Message Data"=w179, "Message"="ReadAcq", "MessageQueue"=w181) -> ("error out"=w178:errorcluster)  [unwired: 7 in, 1 out]
              }
            }
          }
          event User Event {
            n157 = event-data() -> ("ModuleID"=w186:i32, "Data"=w182:variant)  [unwired: 1 in]
            n158 = call <userlib>:"AddressedToThisModule.vi"("ModuleID"=w186, "ModuleAdmin"=w187) -> ("AddressedToThisInstance?"=w185:bool)  [unwired: 8 in, 1 out]
            n159 = case shown="True" w185 {
              tunnel: [_ w188] -> w184
              tunnel: w183 -> [_ w191]
              tunnel: w182 -> [_ w189]
              frame False {
              }
              frame True {
                n160 = call "Enqueue.vi"("Message Data"=w189, "Message"="WriteAcq", "MessageQueue"=w191) -> ("error out"=w188:errorcluster)  [unwired: 7 in, 1 out]
              }
            }
          }
          event User Event {
            n161 = event-data() -> ("ModuleID"=w196:i32, "Data"=w192:variant)  [unwired: 1 in]
            n162 = call <userlib>:"AddressedToThisModule.vi"("ModuleID"=w196, "ModuleAdmin"=w197) -> ("AddressedToThisInstance?"=w195:bool)  [unwired: 8 in, 1 out]
            n163 = case shown="True" w195 {
              tunnel: [_ w198] -> w194
              tunnel: w193 -> [_ w201]
              tunnel: w192 -> [_ w199]
              frame False {
              }
              frame True {
                n164 = call "Enqueue.vi"("Message Data"=w199, "Message"="ConfigAcq", "MessageQueue"=w201) -> ("error out"=w198:errorcluster)  [unwired: 7 in, 1 out]
              }
            }
          }
          event User Event {
            n165 = event-data() -> ("ModuleID"=w206:i32, "Data"=w202:variant)  [unwired: 1 in]
            n166 = call <userlib>:"AddressedToThisModule.vi"("ModuleID"=w206, "ModuleAdmin"=w207) -> ("AddressedToThisInstance?"=w205:bool)  [unwired: 8 in, 1 out]
            n167 = case shown="True" w205 {
              tunnel: [_ w208] -> w204
              tunnel: w203 -> [_ w211]
              tunnel: w202 -> [_ w209]
              frame False {
              }
              frame True {
                n168 = call "Enqueue.vi"("Message Data"=w209, "Message"="ReadTriggers", "MessageQueue"=w211) -> ("error out"=w208:errorcluster)  [unwired: 7 in, 1 out]
              }
            }
          }
          event User Event {
            n169 = event-data() -> ("ModuleID"=w216:i32, "Data"=w212:variant)  [unwired: 1 in]
            n170 = call <userlib>:"AddressedToThisModule.vi"("ModuleID"=w216, "ModuleAdmin"=w217) -> ("AddressedToThisInstance?"=w215:bool)  [unwired: 8 in, 1 out]
            n171 = case shown="True" w215 {
              tunnel: [_ w218] -> w214
              tunnel: w213 -> [_ w221]
              tunnel: w212 -> [_ w219]
              frame False {
              }
              frame True {
                n172 = call "Enqueue.vi"("Message Data"=w219, "Message"="WriteTrigger", "MessageQueue"=w221) -> ("error out"=w218:errorcluster)  [unwired: 7 in, 1 out]
              }
            }
          }
          event User Event {
            n173 = event-data() -> ("ModuleID"=w226:i32, "Data"=w222:variant)  [unwired: 1 in]
            n174 = call <userlib>:"AddressedToThisModule.vi"("ModuleID"=w226, "ModuleAdmin"=w227) -> ("AddressedToThisInstance?"=w225:bool)  [unwired: 8 in, 1 out]
            n175 = case shown="True" w225 {
              tunnel: [_ w228] -> w224
              tunnel: w223 -> [_ w231]
              tunnel: w222 -> [_ w229]
              frame False {
              }
              frame True {
                n176 = call "Enqueue.vi"("Message Data"=w229, "Message"="SyncInfo", "MessageQueue"=w231) -> ("error out"=w228:errorcluster)  [unwired: 7 in, 1 out]
              }
            }
          }
          event User Event {
            n177 = event-data() -> ("ModuleID"=w236:i32, "Data"=w232:variant)  [unwired: 1 in]
            n178 = call <userlib>:"AddressedToThisModule.vi"("ModuleID"=w236, "ModuleAdmin"=w237) -> ("AddressedToThisInstance?"=w235:bool)  [unwired: 8 in, 1 out]
            n179 = case shown="True" w235 {
              tunnel: [_ w238] -> w234
              tunnel: w233 -> [_ w241]
              tunnel: w232 -> [_ w239]
              frame False {
              }
              frame True {
                n180 = call "Enqueue.vi"("Message Data"=w239, "Message"="ConfigTrigger", "MessageQueue"=w241) -> ("error out"=w238:errorcluster)  [unwired: 7 in, 1 out]
              }
            }
          }
          event User Event {
            n181 = event-data() -> ("ModuleID"=w246:i32, "Data"=w242:variant)  [unwired: 1 in]
            n182 = call <userlib>:"AddressedToThisModule.vi"("ModuleID"=w246, "ModuleAdmin"=w247) -> ("AddressedToThisInstance?"=w245:bool)  [unwired: 8 in, 1 out]
            n183 = case shown="True" w245 {
              tunnel: [_ w248] -> w244
              tunnel: w243 -> [_ w251]
              tunnel: w242 -> [_ w249]
              frame False {
              }
              frame True {
                n184 = call "Enqueue.vi"("Message Data"=w249, "Message"="FetchWfrms", "MessageQueue"=w251) -> ("error out"=w248:errorcluster)  [unwired: 7 in, 1 out]
              }
            }
          }
          event User Event {
            n185 = event-data() -> ("ModuleID"=w256:i32, "Data"=w252:variant)  [unwired: 1 in]
            n186 = call <userlib>:"AddressedToThisModule.vi"("ModuleID"=w256, "ModuleAdmin"=w257) -> ("AddressedToThisInstance?"=w255:bool)  [unwired: 8 in, 1 out]
            n187 = case shown="True" w255 {
              tunnel: [_ w258] -> w254
              tunnel: w253 -> [_ w261]
              tunnel: w252 -> [_ w259]
              frame False {
              }
              frame True {
                n188 = call "Enqueue.vi"("Message Data"=w259, "Message"="ReadWfrms", "MessageQueue"=w261) -> ("error out"=w258:errorcluster)  [unwired: 7 in, 1 out]
              }
            }
          }
          event User Event {
            n189 = event-data() -> ("ModuleID"=w266:i32, "Data"=w262:variant)  [unwired: 1 in]
            n190 = call <userlib>:"AddressedToThisModule.vi"("ModuleID"=w266, "ModuleAdmin"=w267) -> ("AddressedToThisInstance?"=w265:bool)  [unwired: 8 in, 1 out]
            n191 = case shown="True" w265 {
              tunnel: [_ w268] -> w264
              tunnel: w263 -> [_ w271]
              tunnel: w262 -> [_ w269]
              frame False {
              }
              frame True {
                n192 = call "Enqueue.vi"("Message Data"=w269, "Message"="Abort", "MessageQueue"=w271) -> ("error out"=w268:errorcluster)  [unwired: 7 in, 1 out]
              }
            }
          }
        }
        n193 = call "ErrorHandler.vi"("error in (no error)"=w44, "MessageQueue"=w42) -> ("error out"=w43:errorcluster)  [unwired: 8 in, 1 out]
      }
    }
    frame Error {
      n194 = property class="ModuleAdmin.lvclass"(reference=w628) -> (reference out=w627:refnum<class "ModuleAdmin.lvclass">, "Accessors:CloneRegRef"=w626:refnum<data-value>, "Accessors:Module ID"=w625:i32)  [unwired: 1 in, 1 out]
      n195 = call <userlib>:"Remove.vi"("Module ID"=w625, "CloneRegRef"=w626) -> ("error out"=w630:errorcluster)  [unwired: 7 in, 2 out]
      n196 = flat-sequence {
        tunnel: w631 -> [w634]
        tunnel: w630 -> [_]
        tunnel: [w632] -> w629
        frame #0 {
          w633 = T10 2 items=["no dialog", "OK message", "continue or stop message", "OK message + warnings", "continue/stop + warnings"] ("type of dialog (OK msg:1)")
          n197 = call <vilib>:"Simple Error Handler.vi"("type of dialog (OK msg:1)"=w633, "error in (no error)"=w634) -> ("error out"=w632:errorcluster)  [unwired: 3 in, 4 out]
        }
      }
    }
  }
  n198 = call "DestroyClone.vi"("error in (no error)"=w15, "Exit via Stop Module Req?"=w11, "Wait for Module to stop?"=w12, "ModuleAdmin"=w13) -> ("error out"=w14:errorcluster, "External Launch"=w10:bool)  [unwired: 5 in, 1 out]
  n199 = Unregister For Events(event registration refnum=w7, error in=w8) -> (error out=w5:errorcluster)
  n200 = Release Queue(queue=w4, force destroy? (F)=FALSE, error in (no error)=w14) -> (error out=w9:errorcluster)  [unwired: 2 out]
  n201 = Merge Errors(w5, w9) -> (w6:errorcluster)
  "error out" <- w6
  n202 = case shown="True" w10 {
    tunnel: w6 -> [_ w636]
    frame False {
    }
    frame True {
      n203 = control-ref of="This VI"() -> (w635:refnum<vi>)
      n204 = case shown="No Error" w636 {
        tunnel: w635 -> [w637 w638]
        frame No Error {
          n205 = invoke class="VI" method="FP.Close"(reference=w637) -> ()  [unwired: 2 in, 3 out]
        }
        frame Error {
          n206 = invoke class="VI" method="FP.Open"(reference=w638, "Activate"=TRUE ("Activate?")) -> ()  [unwired: 3 in, 5 out]
        }
      }
    }
  }
